vi "FTW-ERR-Assert-Truthy.vi"(7 "Assertion":string, 9 "Assertion holds true?":bool, 11 "error in":errorcluster {"code" format="0x%08x (%d)"}) -> (15 "error out":errorcluster {"code" format="0x%08x (%d)"})   [LabVIEW 2015]
panel:
  # "Inputs"
  # "Outputs"
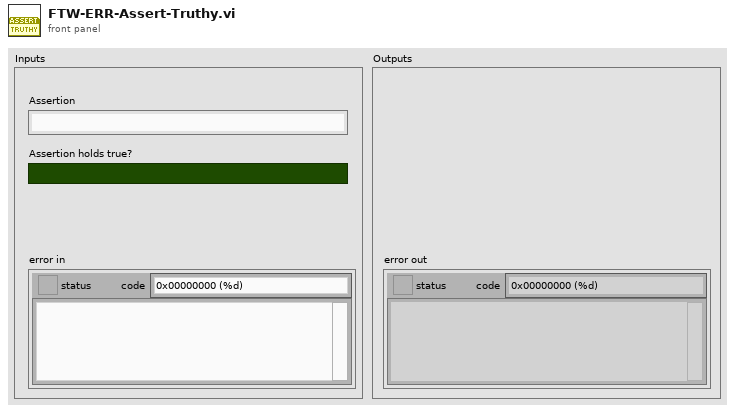
[diagram p1: front panel]
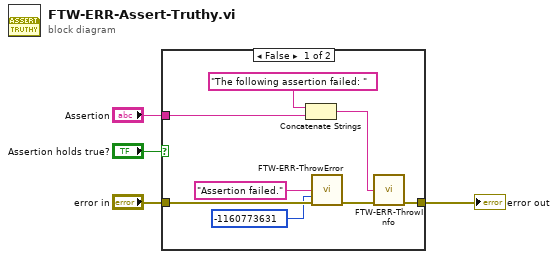
[diagram p0: block diagram]
diagram:
  n1 = case shown="False" "Assertion holds true?" {
    tunnel: "error in" -> [w11 w13]
    tunnel: [w12 w13] -> w3
    tunnel: "Assertion" -> [w7 _]
    frame False {
      n2 = Concatenate Strings("The following assertion failed: " ("string"), w7) -> (w6:string)
      n3 = call "FTW-ERR-ThrowError.vi"("Error Message"="Assertion failed.", "Error Code"=-1160773631, "error in"=w11) -> ("error out"=w10:errorcluster)  [unwired: 12 in]
      n4 = call "FTW-ERR-ThrowInfo.vi"("Informational Message"=w6, "error in"=w10) -> ("error out"=w12:errorcluster)  [unwired: 13 in]
    }
    frame True {
    }
  }
  "error out" <- w3
